vi "Start Channel.vi"(8 "error in":errorcluster, 10 "channel number":u8, 11 "board handle":u8) -> (0 "error out":errorcluster, 2 "channel number out":u8, 3 "board handle out":u8)   [LabVIEW 2020, in "AIM ARINC 429 Hardware API.lvlib"]
uses:
  AIM ARINC 429 Hardware API.lvlib
  Channel Action.ctl
  <instrlib>/AIM GmbH/ARINC-429/subvi/Error Converter (ErrCode or Status).vi
  <instrlib>/AIM GmbH/ARINC-429/subvi/Get Library Path.vi
  <instrlib>/AIM GmbH/ARINC-429/VIs/Library/Api429Lib Error Desc Get.vi
  <instrlib>/AIM GmbH/ARINC-429/subvi/Get Error Number Offset.vi
  <vilib>/Utility/error.llb/Error Cluster From Error Code.vi
  <instrlib>/AIM GmbH/ARINC-429/AIM429LV.lvlib
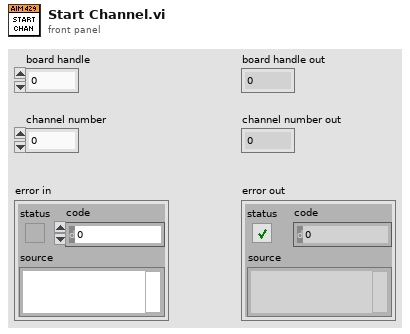
[diagram p1: front panel]
types:
  T1 = typedef "AIM429LV.lvlib/Channel Info Raw.ctl" = cluster{"config_flags":u32, "capability_flags":u32, "speed":u32, "active":u8}
  T2 = typedef "AIM ARINC 429 Hardware API.lvlib/Channel Action.ctl" = enum16{"Get Info", "Initialize", "Start", "Clear"}
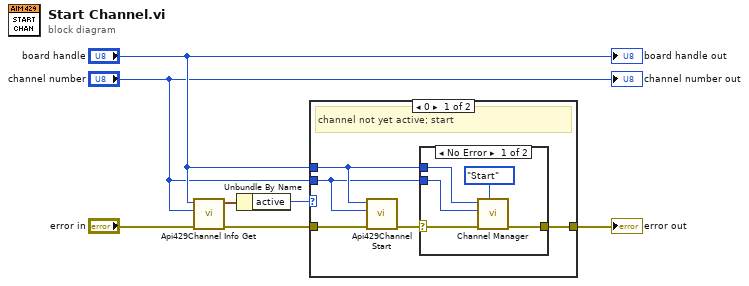
[diagram p0: block diagram]
diagram:
  n1 = call <instrlib>:"Api429Channel Info Get.vi"("error in (no error)"="error in", "channel_id"="channel number", "board_handle"="board handle") -> ("error out"=w4:errorcluster, "pxInfo out"=w6:T1)  [unwired: 7 in]
  n2 = Unbundle By Name(w6) -> ("active"=w3:u8)
  n3 = case shown="0" w3 {
    tunnel: [w11 w19] -> w7
    tunnel: w4 -> [w10 w19]
    tunnel: "board handle" -> [w9 _]
    tunnel: "channel number" -> [w8 _]
    frame 0 {
      # "channel not yet active; start"
      n4 = call <instrlib>:"Api429Channel Start.vi"("error in (no error)"=w10, "channel_id"=w8, "board_handle"=w9) -> ("error out"=w12:errorcluster)  [unwired: 8 in]
      n5 = case shown="No Error" w12 {
        selector: w12 -> [w17 w18]
        tunnel: w9 -> [w15 _]
        tunnel: w8 -> [w16 _]
        tunnel: [w13 w18] -> w11
        frame No Error {
          n6 = call "Channel Manager.vi"("action"=Channel_Action."Start", "error in"=w17, "channel number"=w16, "board handle"=w15) -> ("error out"=w13:errorcluster)  [unwired: 4 in, 3 out]
        }
        frame Error {
        }
      }
    }
    frame Default {
      # "channel already active"
    }
  }
  "error out" <- w7
  "board handle out" <- "board handle"
  "channel number out" <- "channel number"
